vi "VL53L0X_StartMeasurement.vi"(11 "REV2mDistanceSensorDevRef":T1) -> (3 "REV2mDistanceSensorDevRef Out":T1)   [LabVIEW 2019, in "DistanceSensorDriver.lvlib"]
uses:
  DistanceSensorDriver.lvlib
  Typedef/REV2mDistanceSensorDevRef.ctl
  Typedef/Ports.ctl
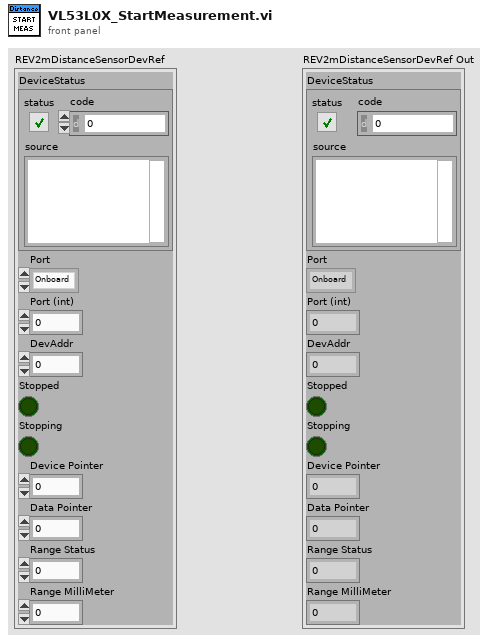
[diagram p1: front panel]
types:
  T1 = typedef "DistanceSensorDriver.lvlib/REV2mDistanceSensorDevRef.ctl" = cluster{"DeviceStatus":errorcluster, "Port":T2, "Port (int)":i32, "DevAddr":i32, "Stopped":bool, "Stopping":bool, "Device Pointer":u64, "Data Pointer":u64, "Range Status":u8, "Range MilliMeter":u16}
  T2 = typedef "DistanceSensorDriver.lvlib/Ports.ctl" = enum32{"Onboard", "MXP"}
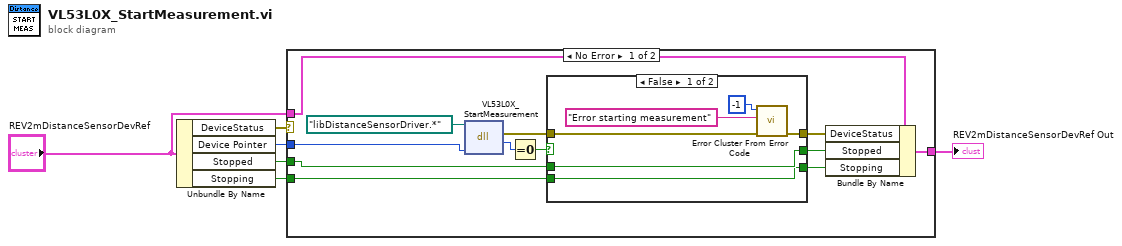
[diagram p0: block diagram]
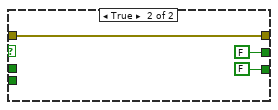
[diagram p2: hidden frame]
diagram:
  n1 = Unbundle By Name("REV2mDistanceSensorDevRef") -> ("DeviceStatus"=w1:errorcluster, "Device Pointer"=w6:u64, "Stopped"=w3:bool, "Stopping"=w2:bool)
  n2 = case shown="No Error" w1 {
    tunnel: w6 -> [w13 _]
    tunnel: [w12 w28] -> w5
    tunnel: "REV2mDistanceSensorDevRef" -> [w11 w28]
    tunnel: w3 -> [w8 _]
    tunnel: w2 -> [w7 _]
    frame No Error {
      n3 = dll-call lib="?" fn="VL53L0X_StartMeasurement"(path in=path "libDistanceSensorDriver.*", "Dev"=w13) -> (error out=w14:errorcluster, "Status"=w15:i32)  [unwired: 3 in, 1 out]
      n4 = Equal To 0?(x=w15) -> (x = 0?=w18:bool)
      n5 = case shown="False" w18 {
        tunnel: w14 -> [w21 w27]
        tunnel: [w24 w27] -> w17
        tunnel: [w20 FALSE ("Stopped")] -> w10
        tunnel: [w19 FALSE ("Stopping")] -> w9
        tunnel: w8 -> [w20 _]
        tunnel: w7 -> [w19 _]
        frame False {
          n6 = call <vilib>:"Error Cluster From Error Code.vi"("error in (no error)"=w21, "error message (\"\")"="Error starting measurement" ("error message (\"\")"), "error code (0)"=-1) -> ("error out"=w24:errorcluster)  [unwired: 6 in]
        }
        frame True {
        }
      }
      n7 = Bundle By Name(cluster=w11, "DeviceStatus"=w17, "Stopped"=w10, "Stopping"=w9) -> (w12:T1)
    }
    frame Error {
    }
  }
  "REV2mDistanceSensorDevRef Out" <- w5
